vi "write_table_mode_command_v2.vi"(10 "Synth Controls":T1={"Channel Settings"=[{"Voltage (Amp.) "=0.0, "Frequency (MHz)"=0.0, "Phase (deg)"=0.0, "Nickname"="Channel 0 D"}, {"Voltage (Amp.) "=0.0, "Frequency (MHz)"=0.0, "Phase (deg)"=0.0, "Nickname"="Channel 0 D"}, {"Voltage (Amp.) "=0.0, "Frequency (MHz)"=0.0, "Phase (deg)"=0.0, "Nickname"="Channel 0 D"}, {"Voltage (Amp.) "=0.0, "Frequency (MHz)"=0.0, "Phase (deg)"=0.0, "Nickname"="Channel 0 D"}], "Active Chans"=[TRUE, FALSE, FALSE, FALSE], "COM Port"="COM5", "Table Mode"={"Initial Frequency (MHz)"=0.0, "FinalFreq"=0.0, "Frequency Step (MHz)"=0.0, "Voltage (Amp.)"=0.0, "Randomize"=FALSE, "Ascending/Descending"=FALSE, "Table Mode Switch"=FALSE}}) -> (2 "Table Mode Command":string)   [LabVIEW 2016]
uses:
  Controls/Synth_409b/Synth_controls.ctl
  Controls/Synth_409b/synth_channel.ctl
  Controls/Synth_409b/table_mode.ctl
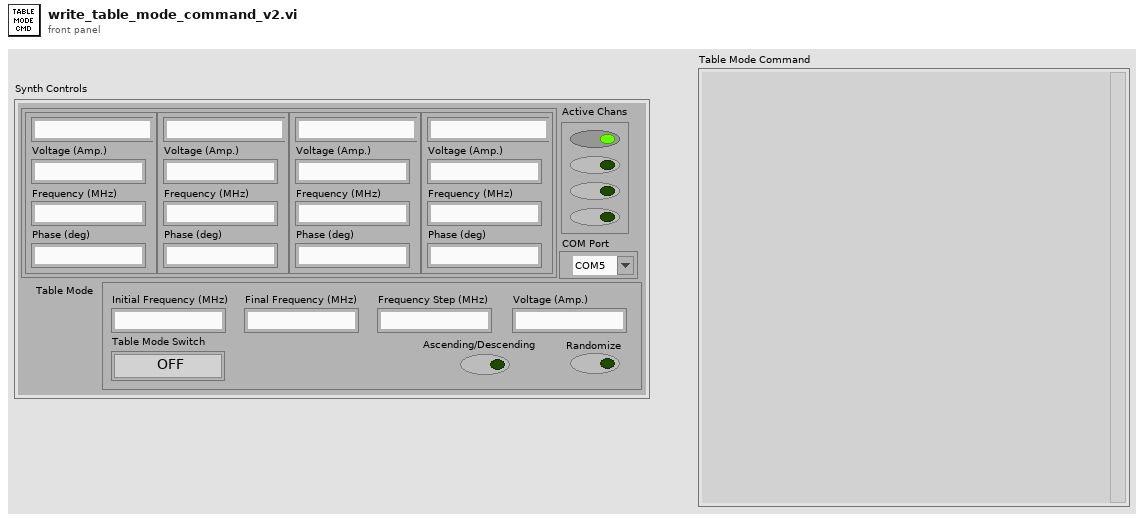
[diagram p1: front panel]
types:
  T1 = typedef "Synth_controls.ctl" = cluster{"Channel Settings":T2[], "Active Chans":bool[], "COM Port":refnum<visa-resource-name>, "Table Mode":T3}
  T2 = typedef "synth_channel.ctl" = cluster{"Voltage (Amp.) ":dbl, "Frequency (MHz)":dbl, "Phase (deg)":dbl, "Nickname":string}
  T3 = typedef "table_mode.ctl" = cluster{"Initial Frequency (MHz)":dbl, "FinalFreq":dbl, "Frequency Step (MHz)":dbl, "Voltage (Amp.)":dbl, "Randomize":bool, "Ascending/Descending":bool, "Table Mode Switch":bool}
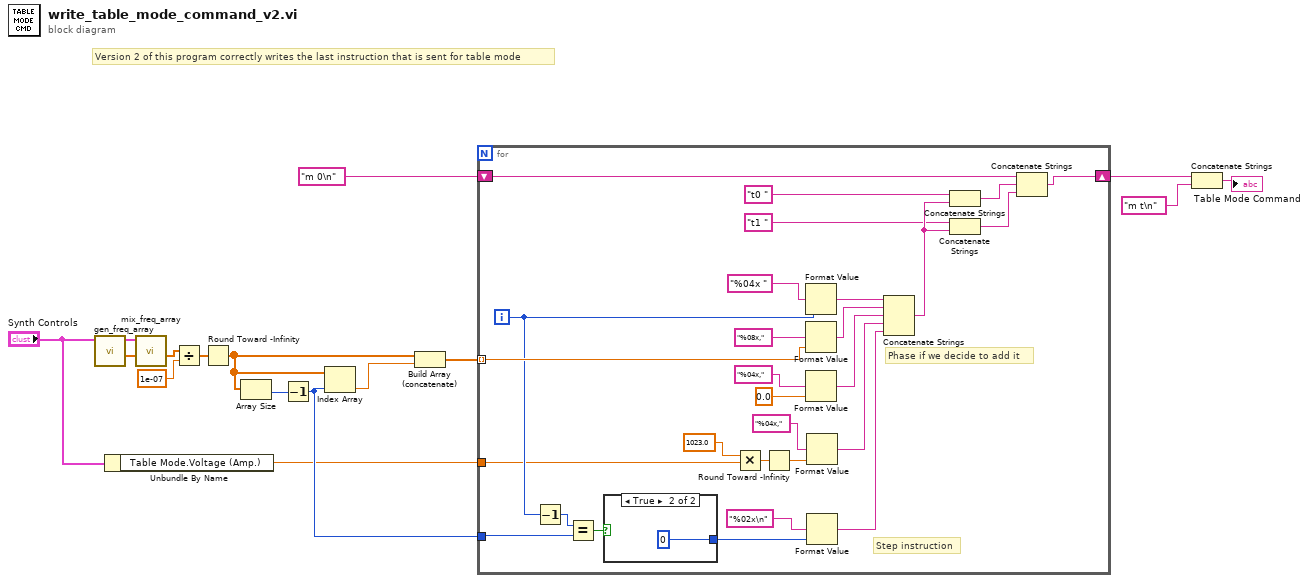
[diagram p0: block diagram]
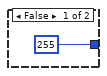
[diagram p2: hidden frame]
diagram:
  # "Version 2 of this program correctly writes the last instruction that is sent for table mode"
  n1 = call "gen_freq_array.vi"("Synth Controls"="Synth Controls") -> ("Synth Controls Out"=w14:T1, "Array"=w15:dbl[])  [unwired: 8 in]
  n2 = Unbundle By Name("Synth Controls") -> ("Table Mode.Voltage (Amp.)"=w1:dbl)
  n3 = call "mix_freq_array.vi"("Freq Array In"=w15, "Synth Controls"=w14) -> ("Mixed Freq Array"=w13:dbl[])  [unwired: 8 in, 1 out]
  n4 = Divide(x=w13, y=1e-07) -> (x/y=w11:dbl[])
  n5 = Round Toward -Infinity(1:w11) -> (0:w6:dbl[])
  n6 = Array Size(array=w6) -> (size(s)=w8:i32)
  n7 = Decrement(x=w8) -> (x-1=w4:i32)
  n8 = Index Array(array=w6, index=w4) -> (element=w7:dbl)
  n9 = Build Array (concatenate)(w6, w7) -> (w5:dbl[])
  n10 = for {
    shift-right: [w34] -> w10
    shift-left: "m 0\n" -> [w33]
    tunnel: w5 -> [w42] mode=indexing
    tunnel: w4 -> [w27]
    tunnel: w1 -> [w17]
    i -> [w23]
    # "Step instruction"
    # "Phase if we decide to add it"
    n11 = Decrement(x=w23) -> (x-1=w24:i32)
    n12 = Equal?(x=w24, y=w27) -> (x = y?=w26:bool)
    n13 = case shown="True" w26 {
      tunnel: [255 0] -> w25
      frame False {
      }
      frame True {
      }
    }
    n14 = Multiply(x=1023.0, y=w17) -> (x*y=w20:dbl)
    n15 = Round Toward -Infinity(1:w20) -> (0:w19:dbl)
    n16 = Format Value(format string="%04x ", value (0)=w23) -> (output string=w43:string)  [unwired: 1 in]
    n17 = Format Value(format string="%08x,", value (0)=w42) -> (output string=w40:string)  [unwired: 1 in]
    n18 = Format Value(format string="%04x,", value (0)=0.0) -> (output string=w37:string)  [unwired: 1 in]
    n19 = Format Value(format string="%04x,", value (0)=w19) -> (output string=w21:string)  [unwired: 1 in]
    n20 = Format Value(format string="%02x\n", value (0)=w25) -> (output string=w35:string)  [unwired: 1 in]
    n21 = Concatenate Strings(w43, w40, w37, w21, w35) -> (w32:string)
    n22 = Concatenate Strings("t0 ", w32) -> (w28:string)
    n23 = Concatenate Strings("t1 ", w32) -> (w29:string)
    n24 = Concatenate Strings(w33, w28, w29) -> (w34:string)
  }
  n25 = Concatenate Strings(w10, "m t\n") -> (→"Table Mode Command":string)
